vi "Assert Member Controller.vi"() -> ()   [LabVIEW 2015, in "Member_Actor.lvlib" / "Member_Actor.lvclass"]
uses:
  Member_Actor.lvclass
  API/_Database/Database.lvclass
  <vilib>/ActorFramework/Actor/Actor.lvclass
panel:
  in  "path":path=path "E:/哈工大竞技机器人队/机器人队管理系统/Database/CRTDatabase.accdb"
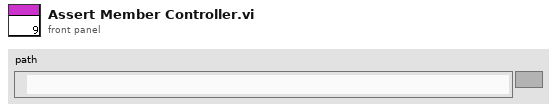
[diagram p1: front panel]
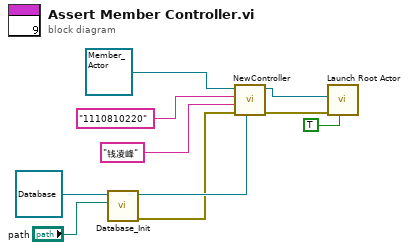
[diagram p0: block diagram]
diagram:
  n1 = call "Database_Init.vi"("path"="path", "object in"=refnum<class "Database.lvclass"> refnum ("Database")) -> ("error out"=w4:errorcluster, "object out"=w5:refnum<class "Database.lvclass">)  [unwired: 8 in]
  n2 = call-dynamic "NewController.vi"("Database"=w5, "error in (no error)"=w4, "Name('')"="钱凌峰", "ID(\"\")"="1110810220" ("ID(\"\")"), "Member_Actor in"=refnum<class "Member_Actor.lvclass"> refnum ("Member_Actor.lvlib:Member_Actor.lvclass")) -> ("error out"=w3:errorcluster, "Member_Actor out"=w2:refnum<class "Member_Actor.lvclass">)  [unwired: 5 in]
  n3 = call <vilib>:"Launch Root Actor.vi"("Open Actor Core front panel? (F)"=TRUE, "error in (no error)"=w3, "Actor"=w2) -> ()  [unwired: 7 in, 2 out]
